vi "XY Graph Register Mouse Move Events.vi"(9 "Error In":errorcluster, 10 "XY Graph Refnum":refnum<vi>) -> (1 "Error Out":errorcluster, 2 "Event Registration Refnum":refnum<event-registration>)   [LabVIEW 2021, in "XY Graph Add-Ons.lvlib"]
doc: "Registers the Enter event for the selected graph, and reserves the Move and Leave events"
uses:
  XY Graph Add-Ons.lvlib
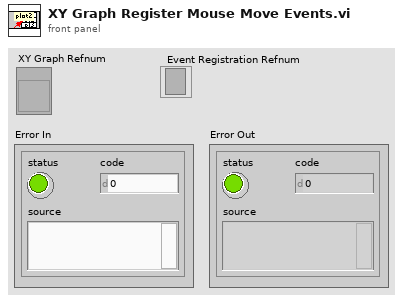
[diagram p1: front panel]
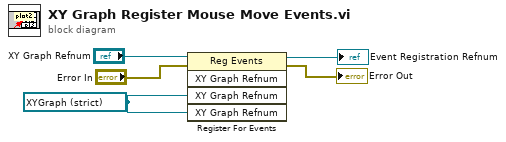
[diagram p0: block diagram]
diagram:
  w4 = refnum<vi> refnum ("XY Graph Refnum")
  n1 = register-events(error in="Error In", "XY Graph Refnum", w4, w4) -> (reference out=→"Event Registration Refnum":refnum<event-registration>, error out=→"Error Out":errorcluster)  [unwired: 1 in]
